vi "highlightAllRows.vi"(8 "error in (no error)":errorcluster, 11 "ScriptEditorV2 in":refnum<class "ScriptEditorV2.lvclass">) -> (0 "error out":errorcluster, 3 "ScriptEditorV2 out":refnum<class "ScriptEditorV2.lvclass">)   [LabVIEW 2011, in "Views.lvlib" / "ScriptEditor.lvlib" / "ScriptEditorV2.lvclass"]
uses:
  ScriptEditorV2.lvclass
  ScriptEditorV2.lvclass/ScriptEditorV2.ctl
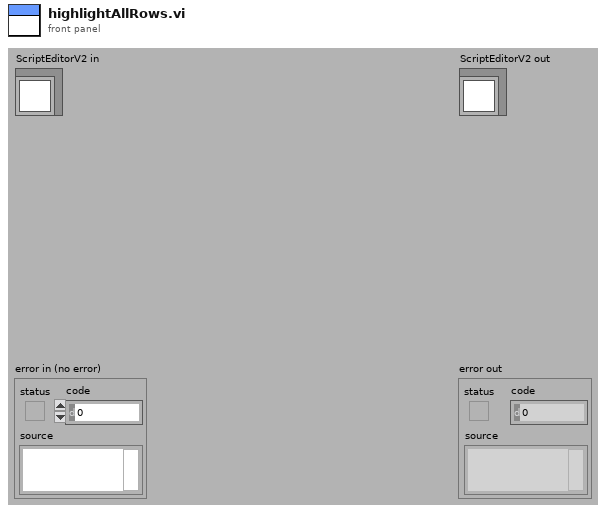
[diagram p1: front panel]
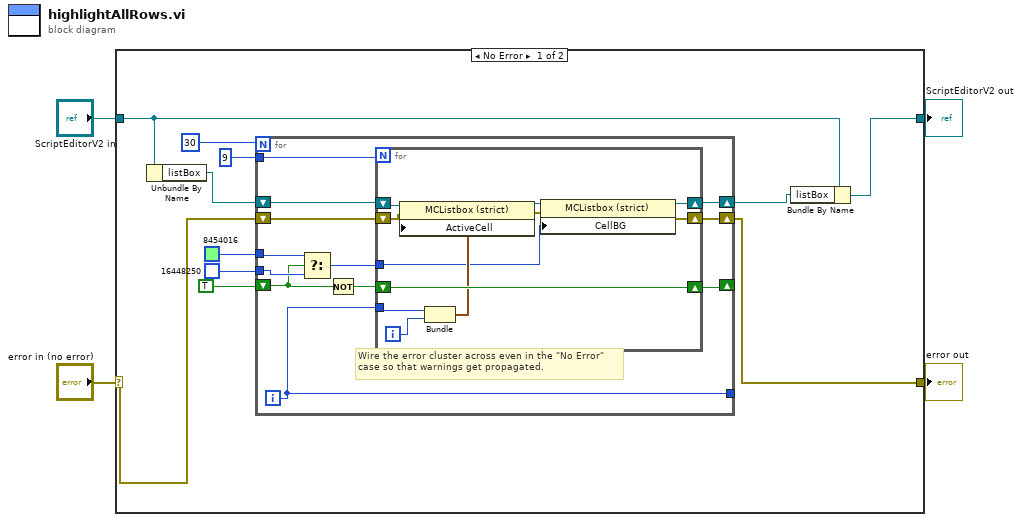
[diagram p0: block diagram]
diagram:
  n1 = case shown="No Error" "error in (no error)" {
    selector: "error in (no error)" -> [w11 w40]
    tunnel: [w10 w40] -> w3
    tunnel: [w7 w39] -> w1
    tunnel: "ScriptEditorV2 in" -> [w8 w39]
    frame No Error {
      # "Wire the error cluster across even in the \"No Error\"\ncase so that warnings get propagated."
      n2 = Unbundle By Name(w8) -> ("listBox"=w12:refnum<vi>)
      n3 = for {
        N: 30 -> [_]
        tunnel: u32 8454016 -> [w24]
        tunnel: u32 16448250 -> [w23]
        tunnel: 9 -> [w27]
        shift-right: [w19] -> _
        shift-left: TRUE -> [w22]
        shift-right: [w18] -> w10
        shift-left: w11 -> [w25]
        shift-right: [w17] -> w9
        shift-left: w12 -> [w26]
        tunnel: [w16] -> _
        i -> [w16]
        n4 = Select(t=w24, s=w22, f=w23) -> (s? t:f=w20:u32)
        n5 = Not(x=w22) -> (.not. x?=w21:bool)
        n6 = for {
          N: w27 -> [_]
          shift-right: [w34] -> w17
          shift-left: w26 -> [w38]
          shift-right: [w33] -> w18
          shift-left: w25 -> [w37]
          shift-right: [w32] -> w19
          shift-left: w21 -> [w32]
          tunnel: w16 -> [w30]
          tunnel: w20 -> [w28]
          i -> [w31]
          n7 = Bundle(w30, w31) -> (w29:cluster{i32, i32})  [unwired: 1 in]
          n8 = property class="MCListbox (strict)"(reference=w38, error in=w37, "ActiveCell"=w29) -> (reference out=w36:refnum<vi>, error out=w35:errorcluster)
          n9 = property class="MCListbox (strict)"(reference=w36, error in=w35, "CellBG"=w28) -> (reference out=w34:refnum<vi>, error out=w33:errorcluster)
        }
      }
      n10 = Bundle By Name(cluster=w8, "listBox"=w9) -> (w7:refnum<class "ScriptEditorV2.lvclass">)
    }
    frame Error {
    }
  }
  "error out" <- w3
  "ScriptEditorV2 out" <- w1
